vi "get Test.vi"(8 "error in (no error)":errorcluster caption="Fehler (Eingang, kein Fehler)", 10 "index":i32 caption="Index", 11 "Report (Eingang)":refnum<class "Report.lvclass">) -> (0 "error out":errorcluster caption="Fehler (Ausgang)", 2 "Test.lvclass":refnum<class "Test.lvclass">, 3 "Report (Ausgang)":refnum<class "Report.lvclass">)   [LabVIEW 2013, in "DatenKlassen.lvlib" / "Report.lvclass"]
uses:
  Report.lvclass
  Test/Test.lvclass
  Report.lvclass/Report.ctl
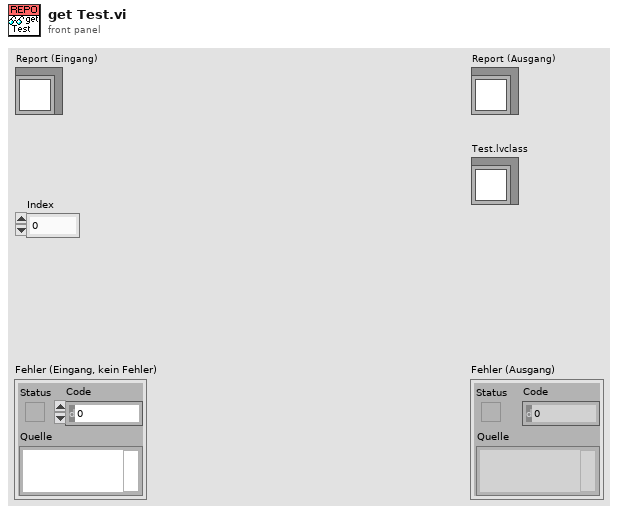
[diagram p1: front panel]
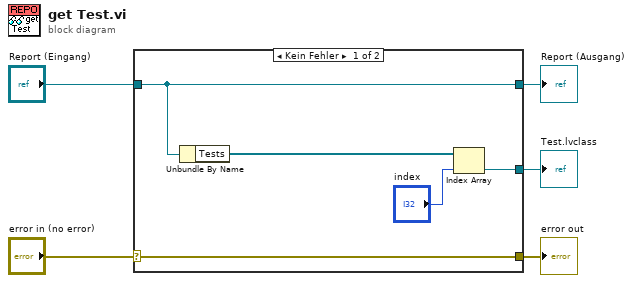
[diagram p0: block diagram]
diagram:
  n1 = case shown="Kein Fehler" "error in (no error)" {
    selector: "error in (no error)" -> [w10 w11]
    tunnel: [w10 w11] -> w4
    tunnel: [w9 w12] -> w2
    tunnel: "Report (Eingang)" -> [w9 w12]
    tunnel: [w6 _] -> w1
    frame No Error {
      n2 = Unbundle By Name(w9) -> ("Tests"=w8:refnum<class "Test.lvclass">[])
      n3 = Index Array(array=w8, index="index") -> (element=w6:refnum<class "Test.lvclass">)
    }
    frame Error {
    }
  }
  "error out" <- w4
  "Report (Ausgang)" <- w2
  "Test.lvclass" <- w1
